vi "Test Timeout Manager.vi"() -> ()   [LabVIEW 2021]
uses:
  Source/Support/Nodes/Leaves/Synch/Parent/WaitOn/bt_WaitOn_Synch.lvclass
  Source/Support/Nodes/Leaves/Synch/Parent/WaitOn/bt_WaitOn_Synch.lvclass/bt_WaitOn_Synch.ctl
  Source/Support/Nodes/Leaves/Synch/Parent/WaitOn/Properties/Write Timeout.vi
panel:
  out "x-y 2":u32
  out "x-y":u32
  out "Timeout Now?":bool
  in  "stop":bool
  out "First Time":bool
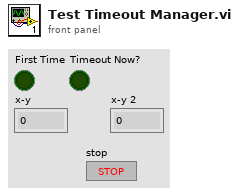
[diagram p1: front panel]
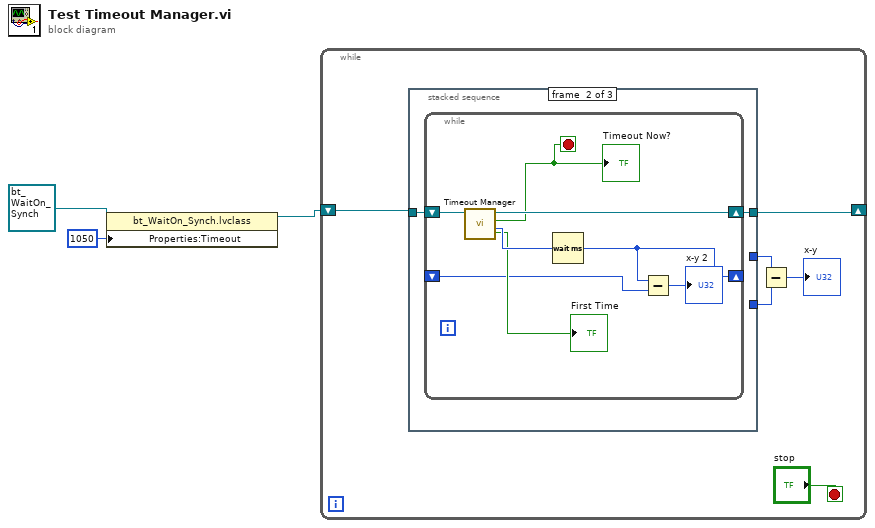
[diagram p0: block diagram]
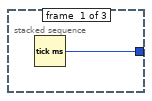
[diagram p2: hidden frame]
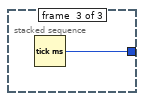
[diagram p3: hidden frame]
diagram:
  n1 = property class="bt_WaitOn_Synch.lvclass"(reference=refnum<class "bt_WaitOn_Synch.lvclass"> refnum ("bt_WaitOn_Synch out"), "Properties:Timeout"=1050 ("Timeout")) -> (reference out=w3:refnum<class "bt_WaitOn_Synch.lvclass">)  [unwired: 1 in, 1 out]
  n2 = while {
    shift-right: [w9] -> _
    shift-left: w3 -> [w8]
    stop <- "stop" stop-if-true
    n3 = stacked-sequence {
      tunnel: [_ w12 _] -> w9
      tunnel: w8 -> [_ w11 _]
      tunnel: [w10 _ _] -> w5
      tunnel: [_ _ w21] -> w6
      frame #0 {
        n4 = Tick Count (ms)() -> (millisecond timer value=w10:u32)
      }
      frame #1 {
        n5 = while {
          shift-right: [w20] -> w12
          shift-left: w11 -> [w19]
          shift-right: [w14] -> _
          shift-left: _ -> [w15]
          stop <- w16 stop-if-true
          n6 = call "Timeout Manager.vi"("bt_WaitOn_Synch in"=w19) -> ("Timeout"=w18:i32, "Timeout Now?"=w16:bool, "bt_WaitOn_Synch out"=w20:refnum<class "bt_WaitOn_Synch.lvclass">, "First Time"=→"First Time":bool)  [unwired: 6 in, 1 out]
          "Timeout Now?" <- w16
          n7 = Wait (ms)(milliseconds to wait=w18) -> (millisecond timer value=w14:u32)
          n8 = Subtract(x=w14, y=w15) -> (x-y=→"x-y 2":u32)
        }
      }
      frame #2 {
        n9 = Tick Count (ms)() -> (millisecond timer value=w21:u32)
      }
    }
    n10 = Subtract(x=w6, y=w5) -> (x-y=→"x-y":u32)
  }
